vi "Save(X,Y,dX,dY)_in_Array-1.vi"(2 "[IN] Array for Replacement":dbl[](array[numeric]), 3 "[IN] Starting Position":i32, 4 "dY":dbl, 5 "dX":dbl, 6 "Y":dbl, 7 "X":dbl) -> (0 "[OUT] Finish Position":i32, 1 "[OUT] Array for Replacement":dbl[](array[numeric]))   [LabVIEW 2017]
doc: "Saving coordinates of displacement into the array"
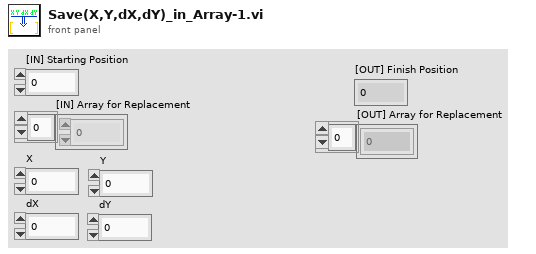
[diagram p1: front panel]
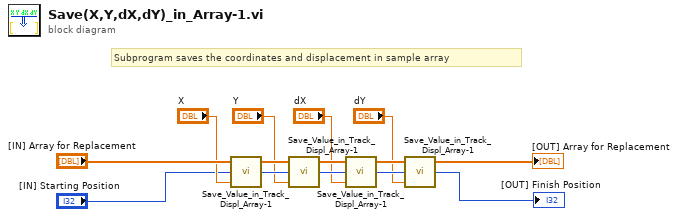
[diagram p0: block diagram]
diagram:
  # "Subprogram saves the coordinates and displacement in sample array"
  n1 = call "Save_Value_in_Track_Displ_Array-1.vi"("[IN] Value"="X", "[IN] Index"="[IN] Starting Position", "[IN] Empty tracks\nfor points saving"="[IN] Array for Replacement") -> ("[OUT] Index ++"=w10:i32, "[OUT Track with saved value"=w11:dbl[])  [unwired: 1 in]
  n2 = call "Save_Value_in_Track_Displ_Array-1.vi"("[IN] Value"="Y", "[IN] Index"=w10, "[IN] Empty tracks\nfor points saving"=w11) -> ("[OUT] Index ++"=w7:i32, "[OUT Track with saved value"=w8:dbl[])  [unwired: 1 in]
  n3 = call "Save_Value_in_Track_Displ_Array-1.vi"("[IN] Value"="dX", "[IN] Index"=w7, "[IN] Empty tracks\nfor points saving"=w8) -> ("[OUT] Index ++"=w4:i32, "[OUT Track with saved value"=w5:dbl[])  [unwired: 1 in]
  n4 = call "Save_Value_in_Track_Displ_Array-1.vi"("[IN] Value"="dY", "[IN] Index"=w4, "[IN] Empty tracks\nfor points saving"=w5) -> ("[OUT] Index ++"=→"[OUT] Finish Position":i32, "[OUT Track with saved value"=→"[OUT] Array for Replacement":dbl[])  [unwired: 1 in]
